vi "ExpEval_ParseInfixToPostfix.vi"(8 "error in (no error)":errorcluster, 11 "infix expression":string) -> (0 "error out":errorcluster, 3 "postfix array":string[](array[string]))   [LabVIEW 2017, in "ExpressionEvaluator.lvlib"]
uses:
  <vilib>/addons/InsightCM/Utilities/ExpressionEvaluator/ExpressionEvaluator.lvlib
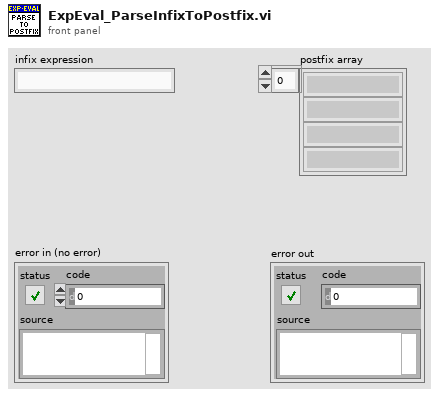
[diagram p1: front panel]
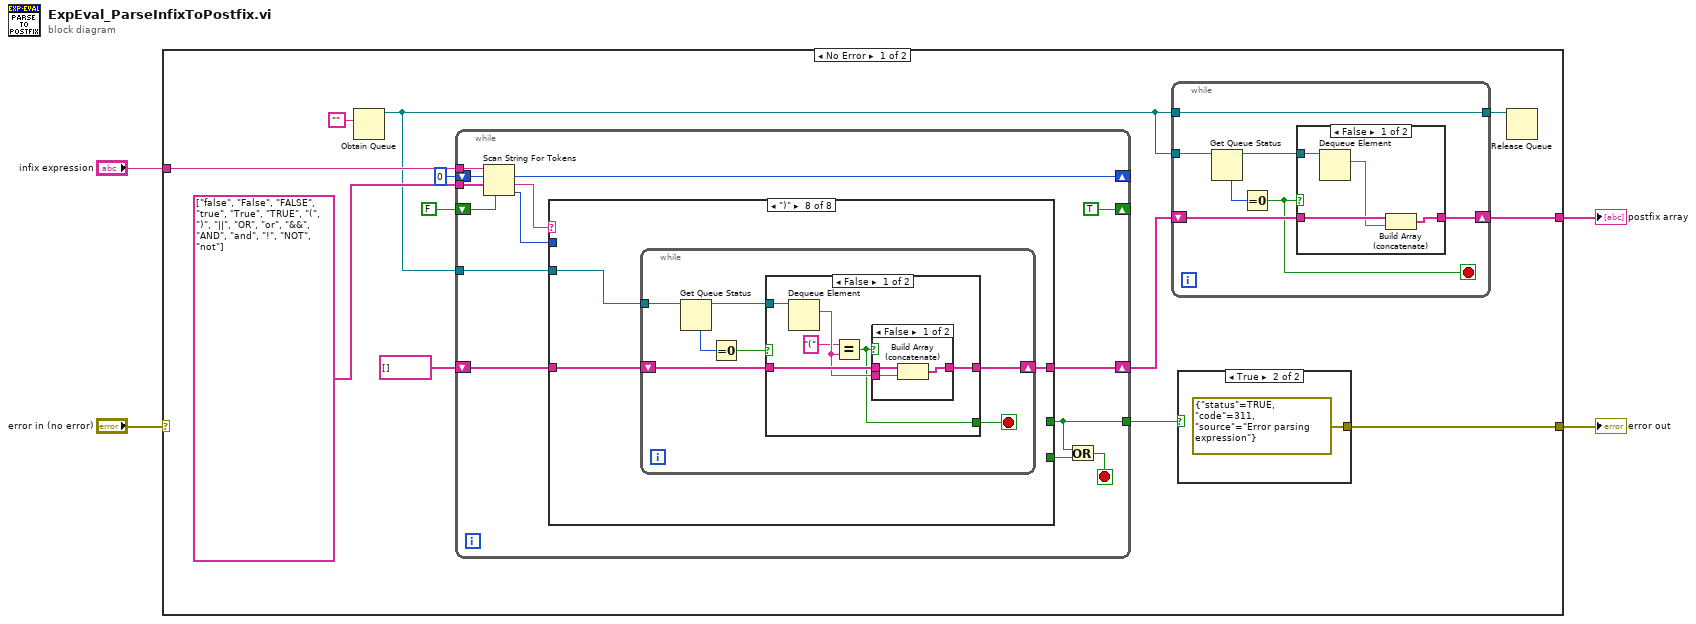
[diagram p0: block diagram]
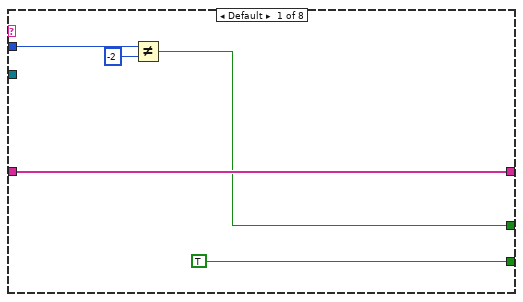
[diagram p4: hidden frame]
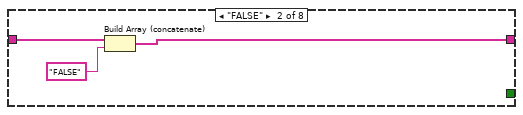
[diagram p5: hidden frame]
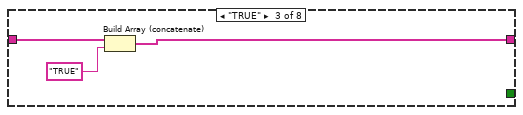
[diagram p6: hidden frame]
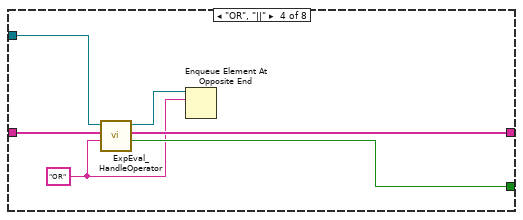
[diagram p7: hidden frame]
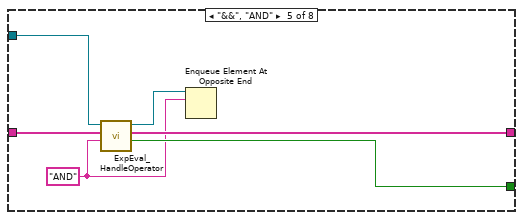
[diagram p8: hidden frame]
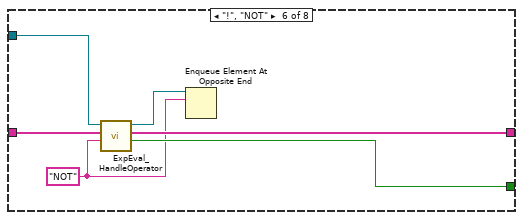
[diagram p9: hidden frame]
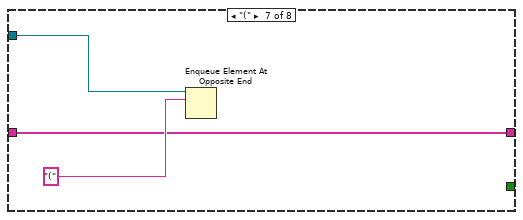
[diagram p10: hidden frame]
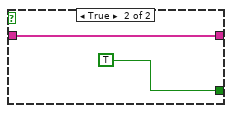
[diagram p12: hidden frame]
diagram:
  n1 = case shown="No Error" "error in (no error)" {
    selector: "error in (no error)" -> [_ w98]
    tunnel: "infix expression" -> [w15 _]
    tunnel: [w11 w98] -> w3
    tunnel: [w8 _] -> w2
    frame No Error {
      n2 = Obtain Queue(element data type="") -> (queue out=w5:refnum<queue>)  [unwired: 4 in, 2 out]
      n3 = while {
        shift-right: [TRUE] -> _
        shift-left: FALSE -> [w43]
        tunnel: string[] ["false", "False", "FALSE", "true", "True", "TRUE", "(", ")", "||", "OR", "or", "&&", "AND", "and", "!", "NOT", "not"] -> [w41]
        tunnel: w15 -> [w40]
        shift-right: [w39] -> _
        shift-left: 0 ("offset past token") -> [w38]
        shift-right: [w37] -> w9
        shift-left: string[] [] ("appended array") -> [w36]
        tunnel: [w34] -> w12
        tunnel: w5 -> [w35]
        stop <- w32 stop-if-true
        n4 = Scan String For Tokens(4:w43, 7:w41, 8:w38, 9:w40) -> (0:w30:i32, 1:w31:string, 2:w39:i32)  [unwired: 2 in, 1 out]
        n5 = case shown="\")\"" w31 {
          tunnel: [w48 w49 w52 w59 w65 w71 w73 w77] -> w37
          tunnel: w36 -> [w48 w51 w54 w60 w66 w72 w73 w78]
          tunnel: [w45 _ _ w58 w64 w70 _ _] -> w34
          tunnel: [TRUE _ _ _ _ _ _ _] -> w33
          tunnel: w35 -> [_ _ _ w56 w62 w68 w74 w76]
          tunnel: w30 -> [w47 _ _ _ _ _ _ _]
          frame Default {
            n6 = Not Equal?(x=w47, y=-2) -> (x != y?=w45:bool)
          }
          frame "FALSE" {
            n7 = Build Array (concatenate)(w51, "FALSE") -> (w49:string[])
          }
          frame "TRUE" {
            n8 = Build Array (concatenate)(w54, "TRUE") -> (w52:string[])
          }
          frame "OR", "||" {
            w57 = "OR"
            n9 = call <vilib>:"ExpEval_HandleOperator.vi"("operator"=w57, "expression in"=w60, "Queue in"=w56) -> ("error"=w58:bool, "expression out"=w59:string[], "Queue out"=w55:refnum<queue>)  [unwired: 6 in]
            n10 = Enqueue Element At Opposite End(queue=w55, element=w57) -> ()  [unwired: 2 in, 3 out]
          }
          frame "&&", "AND" {
            w63 = "AND"
            n11 = call <vilib>:"ExpEval_HandleOperator.vi"("operator"=w63, "expression in"=w66, "Queue in"=w62) -> ("error"=w64:bool, "expression out"=w65:string[], "Queue out"=w61:refnum<queue>)  [unwired: 6 in]
            n12 = Enqueue Element At Opposite End(queue=w61, element=w63) -> ()  [unwired: 2 in, 3 out]
          }
          frame "!", "NOT" {
            w69 = "NOT"
            n13 = call <vilib>:"ExpEval_HandleOperator.vi"("operator"=w69, "expression in"=w72, "Queue in"=w68) -> ("error"=w70:bool, "expression out"=w71:string[], "Queue out"=w67:refnum<queue>)  [unwired: 6 in]
            n14 = Enqueue Element At Opposite End(queue=w67, element=w69) -> ()  [unwired: 2 in, 3 out]
          }
          frame "(" {
            n15 = Enqueue Element At Opposite End(queue=w74, element="(") -> ()  [unwired: 2 in, 3 out]
          }
          frame ")" {
            n16 = while {
              shift-right: [w83] -> w77
              shift-left: w78 -> [w84]
              tunnel: w76 -> [w81]
              stop <- w79 stop-if-true
              n17 = Get Queue Status(queue=w81) -> (queue out=w82:refnum<queue>, # elements in queue=w85:i32)  [unwired: 2 in, 6 out]
              n18 = Equal To 0?(x=w85) -> (x = 0?=w80:bool)
              n19 = case shown="False" w80 {
                tunnel: w82 -> [w91 _]
                tunnel: w84 -> [w90 w97]
                tunnel: [w89 w97] -> w83
                tunnel: [w86 TRUE] -> w79
                frame False {
                  n20 = Dequeue Element(queue=w91) -> (element=w88:string)  [unwired: 2 in, 3 out]
                  n21 = Equal?(x="(", y=w88) -> (x = y?=w86:bool)
                  n22 = case shown="False" w86 {
                    tunnel: w90 -> [w94 w95]
                    tunnel: [w93 w95] -> w89
                    tunnel: w88 -> [w92 _]
                    frame False {
                      n23 = Build Array (concatenate)(w94, w92) -> (w93:string[])
                    }
                    frame True {
                    }
                  }
                }
                frame True {
                }
              }
            }
          }
        }
        n24 = Or(x=w34, y=w33) -> (x .or. y?=w32:bool)
      }
      n25 = while {
        shift-right: [w21] -> w8
        shift-left: w9 -> [w22]
        tunnel: w5 -> [w18]
        tunnel: [w17] -> w6
        tunnel: w5 -> [w17]
        stop <- w19 stop-if-true
        n26 = Get Queue Status(queue=w18) -> (queue out=w20:refnum<queue>, # elements in queue=w23:i32)  [unwired: 2 in, 6 out]
        n27 = Equal To 0?(x=w23) -> (x = 0?=w19:bool)
        n28 = case shown="False" w19 {
          tunnel: w20 -> [w27 _]
          tunnel: w22 -> [w26 w28]
          tunnel: [w24 w28] -> w21
          frame False {
            n29 = Dequeue Element(queue=w27) -> (element=w25:string)  [unwired: 2 in, 3 out]
            n30 = Build Array (concatenate)(w26, w25) -> (w24:string[])
          }
          frame True {
          }
        }
      }
      n31 = case shown="True" w12 {
        tunnel: [_ errorcluster {"status"=TRUE, "code"=311, "source"="Error parsing expression"} ("error constant")] -> w11
        frame False {
        }
        frame True {
        }
      }
      n32 = Release Queue(queue=w6) -> ()  [unwired: 2 in, 3 out]
    }
    frame Error {
    }
  }
  "error out" <- w3
  "postfix array" <- w2
